vi "generator.vi"() -> ()   [LabVIEW 2018]
panel:
  out "error out 2":errorcluster
  out "error out":errorcluster
  in  "Quite":bool
  in  "WriteFiles":bool
  in  "SD Card":path=path "E:/"
  in  "SHT Name":string[](array[string])=["SHT-01", "SHT-02", "SHT-03", "SHT-04", "SHT-05", "SHT-06", "SHT-07", "SHT-08", "SHT-09", "SHT-10", "SHT-11", "SHT-12", "SHT-13", "SHT-14", "SHT-15", "SHT-16"]
  in  "Network select":enum32{"Item 0", "Item 1"}(radio)
  in  "MAC":string="98:76:B6:10:08:d3"
  in  "Mask":string="255.255.255.0"
  in  "Gateway":string="192.168.0.1"
  in  "IP":string="192.168.0.2"
  in  "Password":string="WifiPassword"
  in  "SSID":string="WIFI"
  in  "Box Name":string="Dev"
  # "ESP32 SHT85 Config file editor"
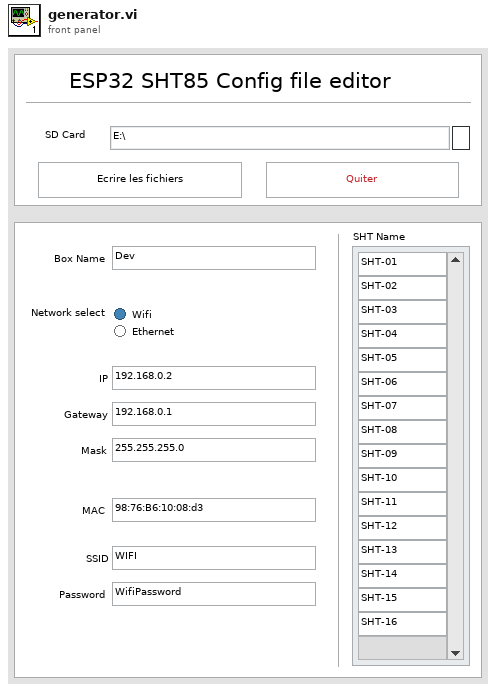
[diagram p1: front panel]
types:
  T1 = enum16{"open", "replace", "create", "open or create", "replace or create", "replace or create with confirmation"}
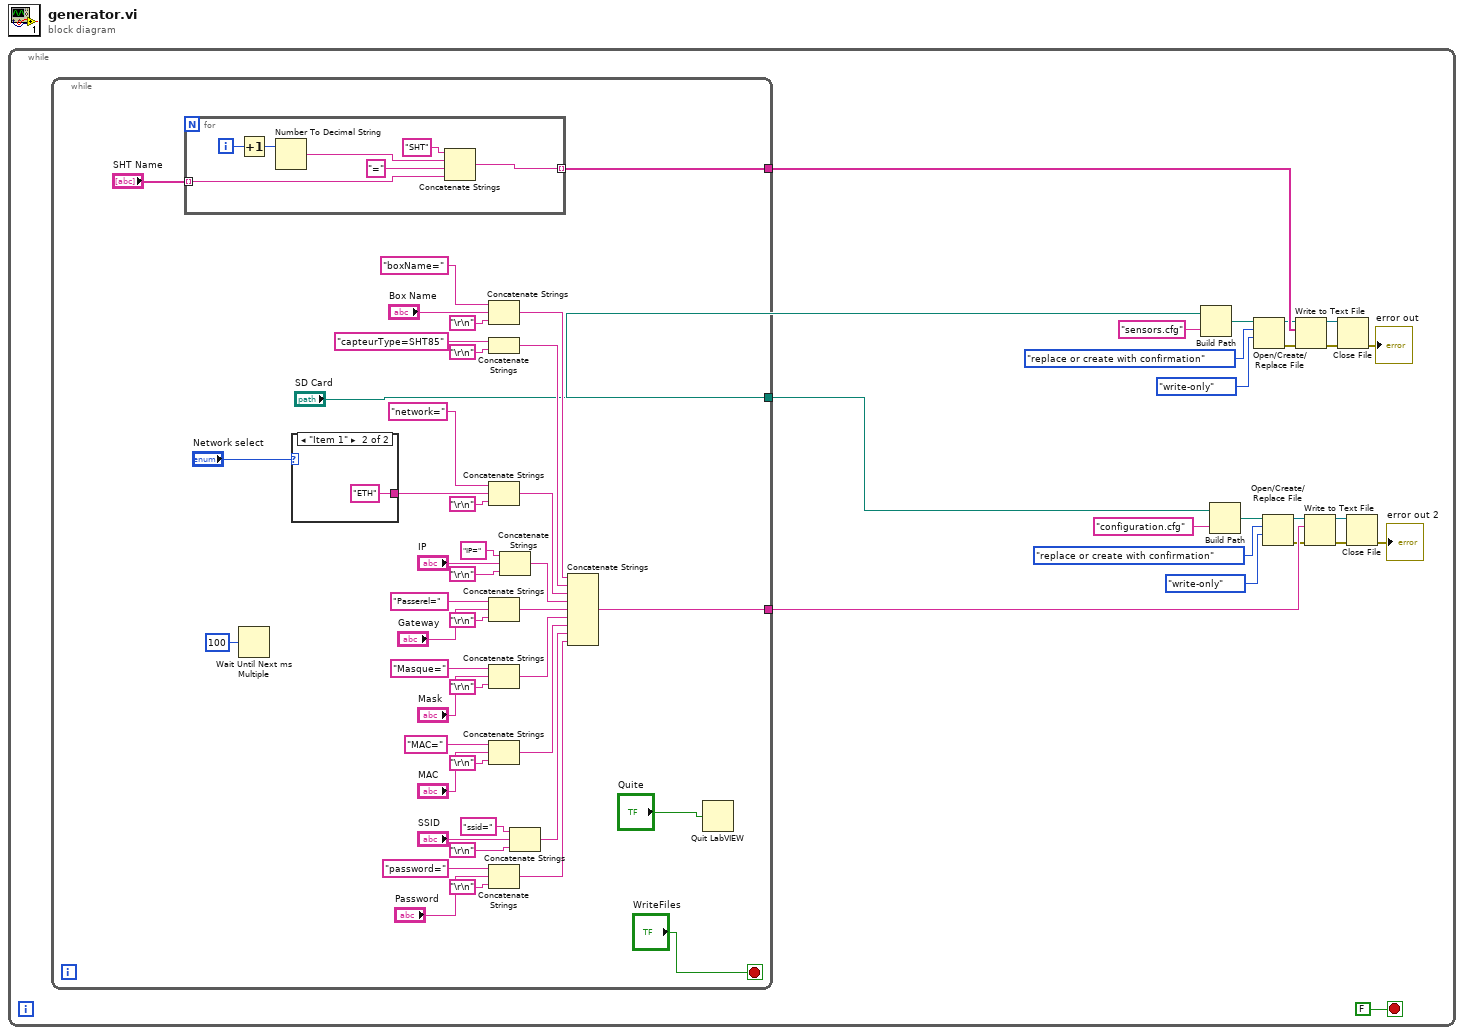
[diagram p0: block diagram]
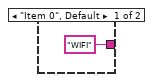
[diagram p2: hidden frame]
diagram:
  n1 = while {
    stop <- FALSE stop-if-true
    n2 = while {
      tunnel: ["SD Card"] -> w20
      tunnel: [w29] -> w13
      tunnel: [w28] -> w12
      stop <- "WriteFiles" stop-if-true
      n3 = for {
        tunnel: "SHT Name" -> [w73] mode=indexing
        tunnel: [w68] -> w28 mode=indexing
        i -> [w72]
        n4 = Increment(x=w72) -> (x+1=w71:i32)
        n5 = Number To Decimal String(number=w71) -> (decimal integer string=w69:string)  [unwired: 1 in]
        n6 = Concatenate Strings("SHT", w69, "=", w73) -> (w68:string)
      }
      n7 = Wait Until Next ms Multiple(millisecond multiple=u32 100) -> ()  [unwired: 1 out]
      n8 = case shown="\"Item 1\"" "Network select" {
        tunnel: ["WIFI" "ETH" ("string")] -> w26
        frame "Item 0", Default {
        }
        frame "Item 1" {
        }
      }
      n9 = Concatenate Strings("boxName=", "Box Name", "\r\n") -> (w46:string)
      n10 = Concatenate Strings("capteurType=SHT85", "\r\n") -> (w45:string)
      n11 = Concatenate Strings("network=", w26, "\r\n") -> (w44:string)
      n12 = Concatenate Strings("Passerel=", "Gateway", "\r\n") -> (w42:string)
      n13 = Concatenate Strings("Masque=", "Mask", "\r\n") -> (w41:string)
      n14 = Concatenate Strings("MAC=", "MAC", "\r\n") -> (w40:string)
      n15 = Concatenate Strings("password=", "Password", "\r\n") -> (w38:string)
      n16 = Concatenate Strings("IP=", "IP", "\r\n") -> (w43:string)
      n17 = Concatenate Strings("ssid=", "SSID", "\r\n") -> (w39:string)
      n18 = Concatenate Strings(w46, w45, w44, w43, w42, w41, w40, w39, w38) -> (w29:string)
      n19 = Quit LabVIEW(quit? (T)="Quite") -> ()
    }
    n20 = Build Path(base path=w20, name or relative path="sensors.cfg") -> (appended path=w22:path)
    n21 = Build Path(base path=w20, name or relative path="configuration.cfg") -> (appended path=w21:path)
    n22 = Open/Create/Replace File(file path (use dialog)=w22, operation (0:open)=T1."replace or create with confirmation", access (0:read/write)=enum16{"read/write", "read-only", "write-only"}."write-only") -> (refnum out=w11:refnum<file>, error out=w4:errorcluster)  [unwired: 3 in, 1 out]
    n23 = Open/Create/Replace File(file path (use dialog)=w21, operation (0:open)=T1."replace or create with confirmation", access (0:read/write)=enum16{"read/write", "read-only", "write-only"}."write-only") -> (refnum out=w10:refnum<file>, error out=w5:errorcluster)  [unwired: 3 in, 1 out]
    n24 = Write to Text File(file (use dialog)=w11, text=w12, error in=w4) -> (refnum out=w8:refnum<file>, error out=w9:errorcluster)  [unwired: 1 in, 1 out]
    n25 = Write to Text File(file (use dialog)=w10, text=w13, error in=w5) -> (refnum out=w6:refnum<file>, error out=w7:errorcluster)  [unwired: 1 in, 1 out]
    n26 = Close File(refnum=w8, error in=w9) -> (error out=→"error out":errorcluster)  [unwired: 1 out]
    n27 = Close File(refnum=w6, error in=w7) -> (error out=→"error out 2":errorcluster)  [unwired: 1 out]
  }
